vi "动态调用可重入VI.vi"() -> ()   [LabVIEW 2013]
panel:
  out "可重入？":bool[](array[boolean])
  out "VI副本名称":string[](array[string])
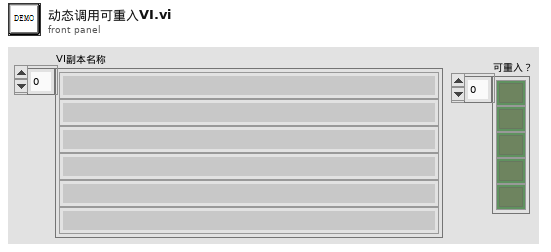
[diagram p1: front panel]
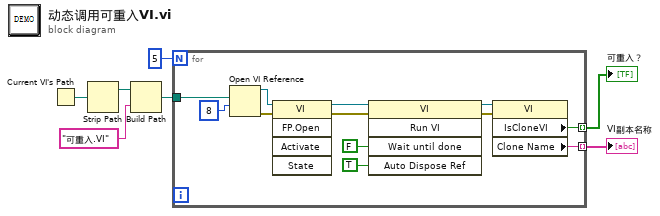
[diagram p0: block diagram]
diagram:
  n1 = Current VI's Path() -> (path=w6:path)
  n2 = Strip Path(path=w6) -> (stripped path=w5:path)  [unwired: 1 out]
  n3 = Build Path(base path=w5, name or relative path="可重入.VI" ("名称或相对路径")) -> (appended path=w3:path)
  n4 = for {
    N: 5 -> [_]
    tunnel: w3 -> [w18]
    tunnel: [w9] -> w2 mode=indexing
    tunnel: [w8] -> w1 mode=indexing
    n5 = Open VI Reference(vi path=w18, options=8 ("选项")) -> (vi reference=w17:refnum<vi>, error out=w16:errorcluster)  [unwired: 4 in]
    n6 = invoke class="VI" method="FP.Open"(reference=w17, error in=w16) -> (reference out=w15:refnum<vi>, error out=w14:errorcluster)  [unwired: 3 in, 3 out]
    n7 = invoke class="VI" method="Run VI"(reference=w15, error in=w14, "Wait until done"=FALSE ("结束前等待"), "Auto Dispose Ref"=TRUE ("自动销毁引用")) -> (reference out=w11:refnum<vi>, error out=w10:errorcluster)  [unwired: 1 in, 3 out]
    n8 = property class="VI"(reference=w11, error in=w10) -> ("IsCloneVI"=w9:bool, "Clone Name"=w8:string)  [unwired: 2 out]
  }
  "VI副本名称" <- w1
  "可重入？" <- w2
